vi "OpenCL Test.vi"(11 "Init":bool) -> (0 "DLL To Use":path)   [LabVIEW 2012, in "OpenCLV x64.lvlib"]
uses:
  OpenCLV x64.lvlib
  <vilib>/Utility/sysdir.llb/System Directory Type.ctl
panel:
  out "Application:Directory Path":path
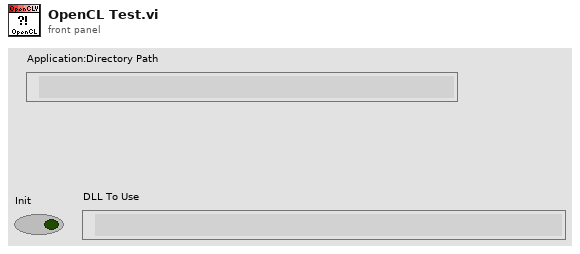
[diagram p1: front panel]
types:
  T1 = typedef "System Directory Type.ctl" = i32
  T2 = enum32{"invalid app kind", "Development System", "Run Time System", "Student Edition", "Embedded LabVIEW", "Evaluation", "Custom"}
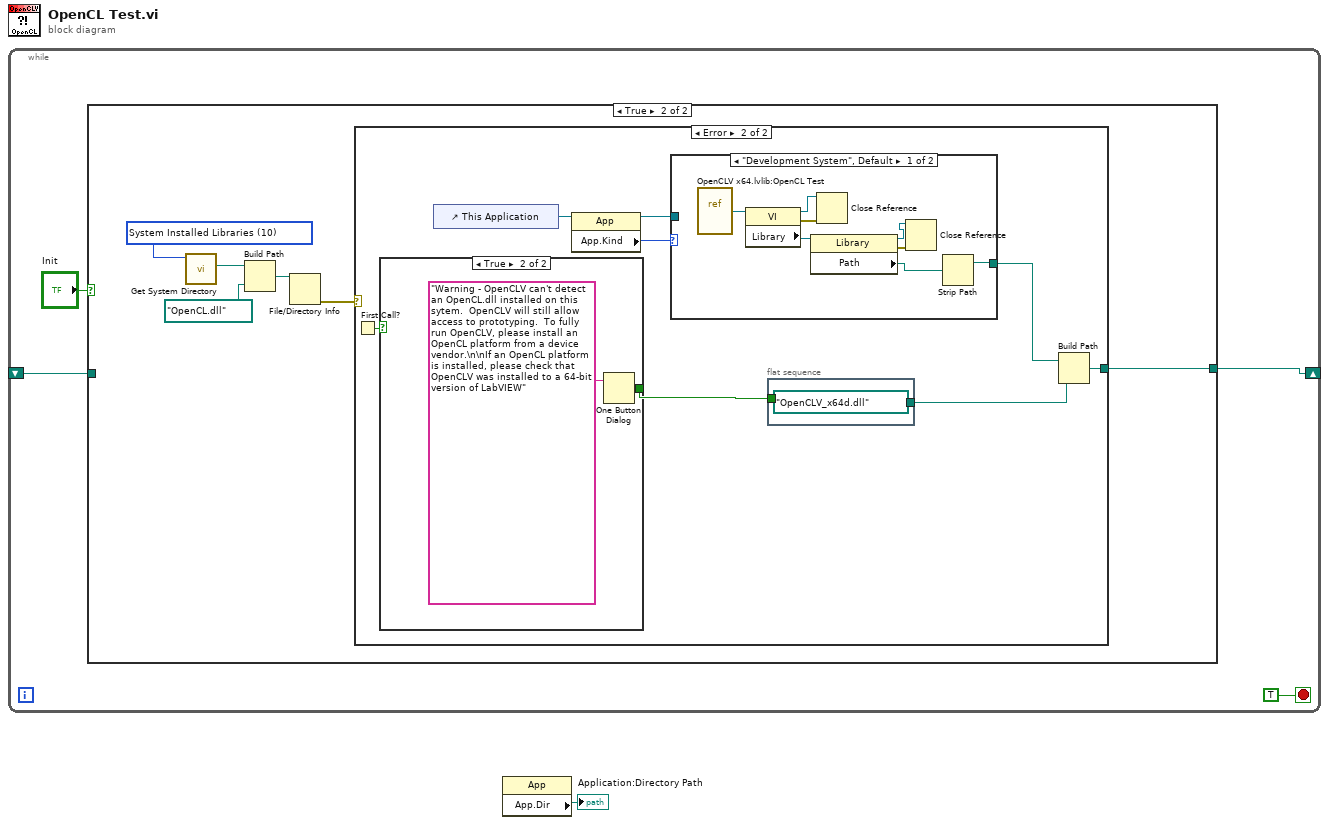
[diagram p0: block diagram]
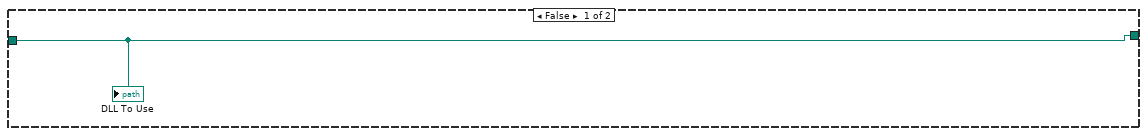
[diagram p2: hidden frame]
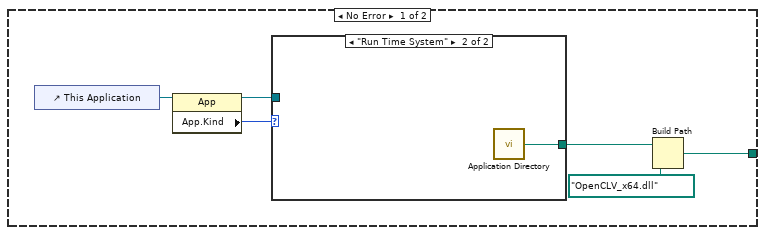
[diagram p3: hidden frame]
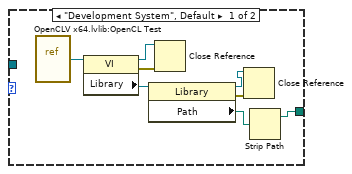
[diagram p4: hidden frame]
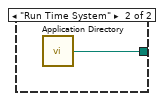
[diagram p5: hidden frame]
diagram:
  n1 = while {
    shift-right: [w5] -> _
    shift-left: _ -> [w4]
    stop <- TRUE stop-if-true
    n2 = case shown="True" "Init" {
      tunnel: [w6 w8] -> w5
      tunnel: w4 -> [w6 _]
      frame False {
        "DLL To Use" <- w6
      }
      frame True {
        w12 = T1 10 items=["User Home"=0, "User Desktop"=1, "User Documents"=2, "User Application Data"=3, "User Preferences"=4, "User Temporary"=5, "Public Documents"=6, "Public Application Data"=7, "Public Preferences"=8, "Public Cache"=13, "System Core Libraries"=9, "System Installed Libraries"=10, "Application Files"=11, "Boot Volume Root"=12] ("system directory type")
        n3 = call <vilib>:"Get System Directory.vi"("system directory type"=w12) -> ("system directory"=w11:path)  [unwired: 10 in]
        n4 = Build Path(base path=w11, name or relative path=path "OpenCL.dll" ("path")) -> (appended path=w9:path)
        n5 = File/Directory Info(path=w9) -> (error out=w7:errorcluster)  [unwired: 1 in, 6 out]
        n6 = case shown="Error" w7 {
          tunnel: [w17 w34] -> w8
          frame No Error {
            n7 = control-ref of="This Application"() -> (w16:refnum<vi>)
            n8 = property class="App"(reference=w16) -> (reference out=w13:refnum<vi>, "App.Kind"=w15:T2)  [unwired: 1 in, 1 out]
            n9 = case shown="\"Run Time System\"" w15 {
              tunnel: [w19 w27] -> w14
              tunnel: w13 -> [_ _]
              frame "Development System", Default {
                n10 = vi-ref "OpenCLV x64.lvlib:OpenCL Test.vi"() -> (w26:refnum<vi>)
                n11 = property class="VI"(reference=w26) -> (reference out=w21:refnum<vi>, error out=w22:errorcluster, "Library"=w25:refnum<vi>)  [unwired: 1 in]
                n12 = property class="Library"(reference=w25) -> (reference out=w23:refnum<vi>, error out=w24:errorcluster, "Path"=w20:path)  [unwired: 1 in]
                n13 = Close Reference(reference=w21, error in (no error)=w22) -> ()  [unwired: 1 out]
                n14 = Close Reference(reference=w23, error in (no error)=w24) -> ()  [unwired: 1 out]
                n15 = Strip Path(path=w20) -> (stripped path=w19:path)  [unwired: 1 out]
              }
              frame "Run Time System" {
                n16 = call <vilib>:"Application Directory.vi"() -> ("Application Directory"=w27:path)
              }
            }
            n17 = Build Path(base path=w14, name or relative path=path "OpenCLV_x64.dll" ("path")) -> (appended path=w17:path)
          }
          frame Error {
            n18 = First Call?() -> (First Call?: T/F=w33:bool)
            n19 = case shown="True" w33 {
              selector: w33 -> [w45 _]
              tunnel: [w45 w47] -> w32
              frame False {
              }
              frame True {
                n20 = One Button Dialog(message="Warning - OpenCLV can't detect an OpenCL.dll installed on this sytem.  OpenCLV will still allow access to prototyping.  To fully run OpenCLV, please install an OpenCL platform from a device vendor.\n\nIf an OpenCL platform is installed, please check that OpenCLV was installed to a 64-bit version of LabVIEW") -> (true=w47:bool)  [unwired: 1 in]
              }
            }
            n21 = control-ref of="This Application"() -> (w31:refnum<vi>)
            n22 = property class="App"(reference=w31) -> (reference out=w29:refnum<vi>, "App.Kind"=w30:T2)  [unwired: 1 in, 1 out]
            n23 = case shown="\"Development System\", Default" w30 {
              tunnel: [w37 w44] -> w28
              tunnel: w29 -> [_ _]
              frame "Development System", Default {
                n24 = vi-ref "OpenCLV x64.lvlib:OpenCL Test.vi"() -> (w43:refnum<vi>)
                n25 = property class="VI"(reference=w43) -> (reference out=w38:refnum<vi>, error out=w39:errorcluster, "Library"=w42:refnum<vi>)  [unwired: 1 in]
                n26 = property class="Library"(reference=w42) -> (reference out=w40:refnum<vi>, error out=w41:errorcluster, "Path"=w36:path)  [unwired: 1 in]
                n27 = Close Reference(reference=w38, error in (no error)=w39) -> ()  [unwired: 1 out]
                n28 = Close Reference(reference=w40, error in (no error)=w41) -> ()  [unwired: 1 out]
                n29 = Strip Path(path=w36) -> (stripped path=w37:path)  [unwired: 1 out]
              }
              frame "Run Time System" {
                n30 = call <vilib>:"Application Directory.vi"() -> ("Application Directory"=w44:path)
              }
            }
            n31 = flat-sequence {
              tunnel: [path "OpenCLV_x64d.dll" ("path")] -> w35
              tunnel: w32 -> [_]
              frame #0 {
              }
            }
            n32 = Build Path(base path=w28, name or relative path=w35) -> (appended path=w34:path)
          }
        }
      }
    }
  }
  n33 = property class="App"() -> ("App.Dir"=→"Application:Directory Path":path)  [unwired: 2 in, 2 out]
